vi "uTTA_GV_Serial_Monitor.vi"() -> ()   [LabVIEW 2021]
panel:
  in  "Buffer Length":u32=2048
  out "Enabled":bool
  out "Serial Monitor":string="*IDN?\nSYST:MODE CAL\nSYST:RATE 25\nMEAS:SET ISEN,0.000000\nMEAS:SET ISEN,4095.000000\nMEAS:SET ISEN,8190.000000\nMEAS:SET ISEN,12285.000000\nMEAS:SET ISEN,16380.000000\nMEAS:SET ISEN,20475.000000\nMEAS:SET ISEN,24570.000000\nMEAS:SET ISEN,28665.000000\nMEAS:SET ISEN,32760.000000\nMEAS:SET ISEN,36855.000000\nMEAS:SET ISEN,40950.000000\nMEAS:SET ISEN,45045.000000\nMEAS:SET ISEN,49140.000000\nMEAS:SET ISEN,53235.000000\nMEAS:SET ISEN,57330.000000\nMEAS:SET ISEN,61425.000000\nMEAS:SET ISEN,65520.000000\nMEAS:SET ISEN,0.000000\nMEAS:STOP\n*IDN?\n*** DEBUG INFO ***\nTOKENS: 31\n    *IDN\n    *RST\n    *ESR\n    *STB\n    MEMory\n    READfile\n    WRITEtest\n    DIRectory\n    DELete\n    UPLoad\n    MEASure\n    TIMe\n    PREheating\n    HEATing\n    COOLing\n    START\n    STOP\n    DUT\n    CHDESCription\n    SET\n    SYSTem\n    MODE\n    RATE\n    GAIN\n    CAL\n    SAVE\n    PSUenable\n    POWERstage\n    GDPOWer\n    PWUVlo\n    CLOCK\n\nVALID CODES: 36\n   234\n   160\n   84\n   137\n   196\n   197\n   198\n   199\n   200\n   180\n   67\n   181\n   120\n   182\n   173\n   167\n   12\n   13\n   14\n   15\n   16\n   36\n   37\n   38\n   221\n   39\n   40\n   41\n   124\n   42\n   177\n   43\n   230\n   27\n   80\n   45\n\n*******************\nInit SD Card!\nW25QXX successfully initialized\nManufacturer       = 0xef\nDevice             = 0x4018\nBlock size         = 0x10000 (65536)\nBlock count        = 0x0100 (256)\nTotal size (in kB) = 0x4000 (16384)\nLittleFS Init\nError 3.003\nDAC Initialisation!\nInit completed!\nRTC Time: 21.10.2024 22:26:25\n*** DEBUG INFO ***\nTOKENS: 31\n    *IDN\n    *RST\n    *ESR\n    *STB\n    MEMory\n    READfile\n    WRITEtest\n    DIRectory\n    DELete\n    UPLoad\n    MEASure\n    TIMe\n    PREheating\n    HEATing\n    COOLing\n    START\n    STOP\n    DUT\n    CHDESCription\n    SET\n    SYSTem\n    MODE\n    RATE\n    GAIN\n    CAL\n    SAVE\n    PSUenable\n    POWERstage\n    GDPOWer\n    PWUVlo\n    CLOCK\n\nVALID CODES: 36\n   234\n   160\n   84\n   137\n   196\n   197\n   198\n   199\n   200\n   180\n   67\n   181\n   120\n   182\n   173\n   167\n   12\n   13\n   14\n   15\n   16\n   36\n   37\n   38\n   221\n   39\n   40\n   41\n   124\n   42\n   177\n   43\n   230\n   27\n   80\n   45\n\n*******************\nInit SD Card!\nW25QXX successfully initialized\nManufacturer       = 0xef\nDevice             = 0x4018\nBlock size         = 0x10000 (65536)\nBlock count        = 0x0100 (256)\nTotal size (in kB) = 0x4000 (16384)\nLittleFS Init\nError 3.003\nDAC Initialisation!\nInit completed!\nRTC Time: 21.10.2024 22:26:28\n*IDN?\nWK, uTTA, SN001, 2.0, Oct 21 2024, 19:46:16\nSYST:MODE CAL\nOK\nSYST:RATE 25\n25\nMEAS:SET ISEN,0.000000\nOK 2\nMEAS:SET ISEN,4095.000000\nOK 2\nMEAS:SET ISEN,8190.000000\nOK 2\nMEAS:SET ISEN,12285.000000\nOK 2\nMEAS:SET ISEN,16380.000000\nOK 2\nMEAS:SET ISEN,20475.000000\nOK 2\nMEAS:SET ISEN,24570.000000\nOK 2\nMEAS:SET ISEN,28665.000000\nOK 2\nMEAS:SET ISEN,32760.000000\nOK 2\nMEAS:SET ISEN,36855.000000\nOK 2\nMEAS:SET ISEN,40950.000000\nOK 2\nMEAS:SET ISEN,45045.000000\nOK 2\nMEAS:SET ISEN,49140.000000\nOK 2\nMEAS:SET ISEN,53235.000000\nOK 2\nMEAS:SET ISEN,57330.000000\nOK 2\nMEAS:SET ISEN,61425.000000\nOK 2\nMEAS:SET ISEN,65520.000000\nOK 2\nMEAS:SET ISEN,0.000000\nOK 2\nMEAS:START\nOK\nMEAS:SET VOFF0,0.000000\nMEAS:SET VOFF0,4095.000000\nMEAS:SET VOFF0,8190.000000\nMEAS:SET VOFF0,12285.000000\nMEAS:SET VOFF0,16380.000000\n"
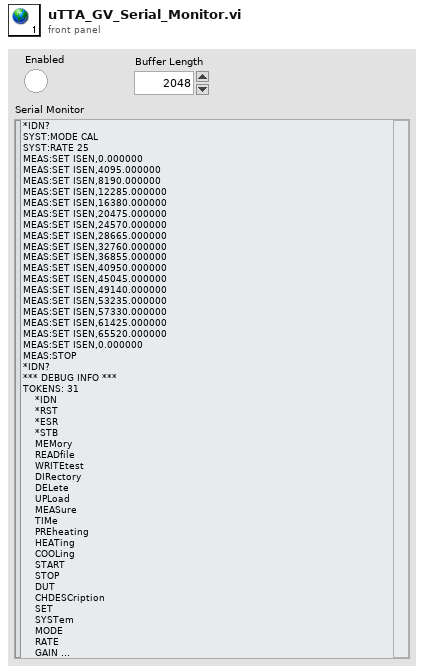
[diagram p1: front panel]
diagram:
